vi "pueba.vi"(0 "Ruta":path, 3 "Método":enum16{"G", "Gx", "Gy"}(ring)) -> ()   [LabVIEW 2020]
doc: "Ceballos Conde Emanuel 4MV6 Sistemas de visión artificial 2022/1\nEste vi permite obtener el gradiente en x , gradiente en Y o gradiente general en susecion de una serie de imagenes ubicadas en una carpeta , si se utiliza como subvi la salida obtenida sera el gradiente da la ultima imagen de la carpeta."
panel:
  out "Bcx":u32
  out "Bcy":u32
  out "Gcx":u32
  out "Gcy":u32
  out "Rcy":u32
  out "Rcx":u32
  out "Image":T1(plugin-control)
  # "Ceballos Conde Emanuel\n4MV6\nSistemas de visión artificial\n2022/1"
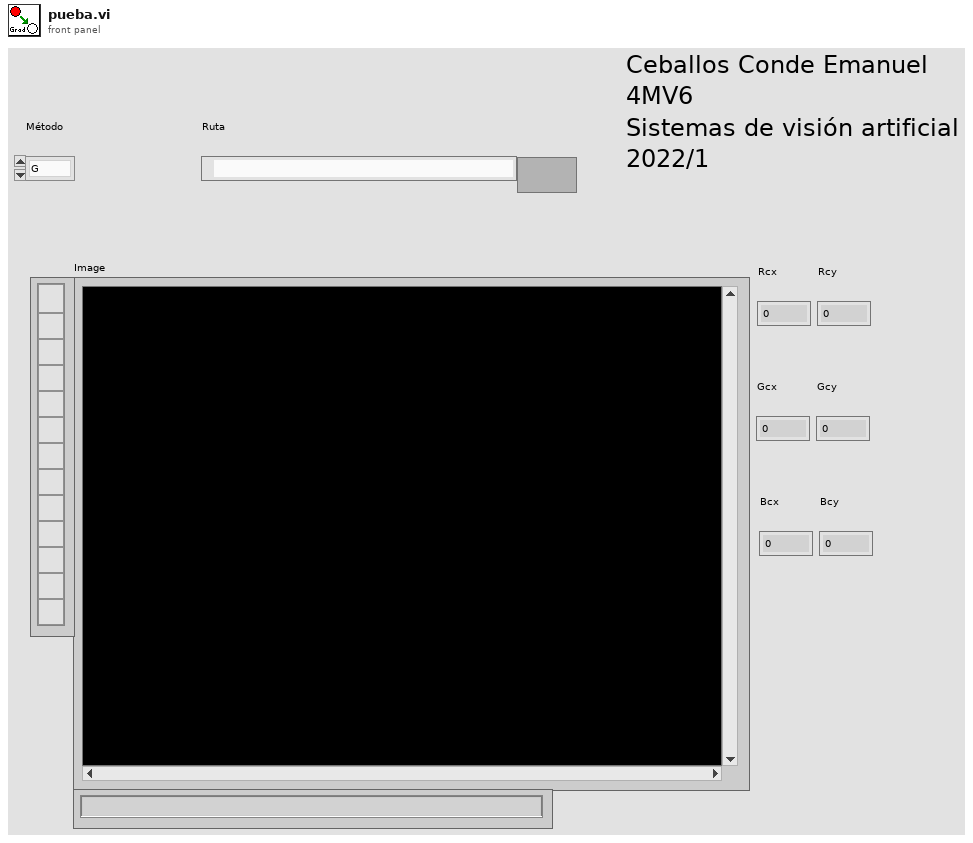
[diagram p1: front panel]
types:
  T1 = typedef "IMAQ Image.ctl" = refnum<image>
  T2 = typedef "Image Type" = u32
  T3 = typedef "imagedata.ctl" = cluster{"image type":i32, "image depth":i32, "image":u8[], "mask":u8[], "colors":u32[], "Rectangle":cluster{"left":i16, "top":i16, "right":i16, "bottom":i16}}
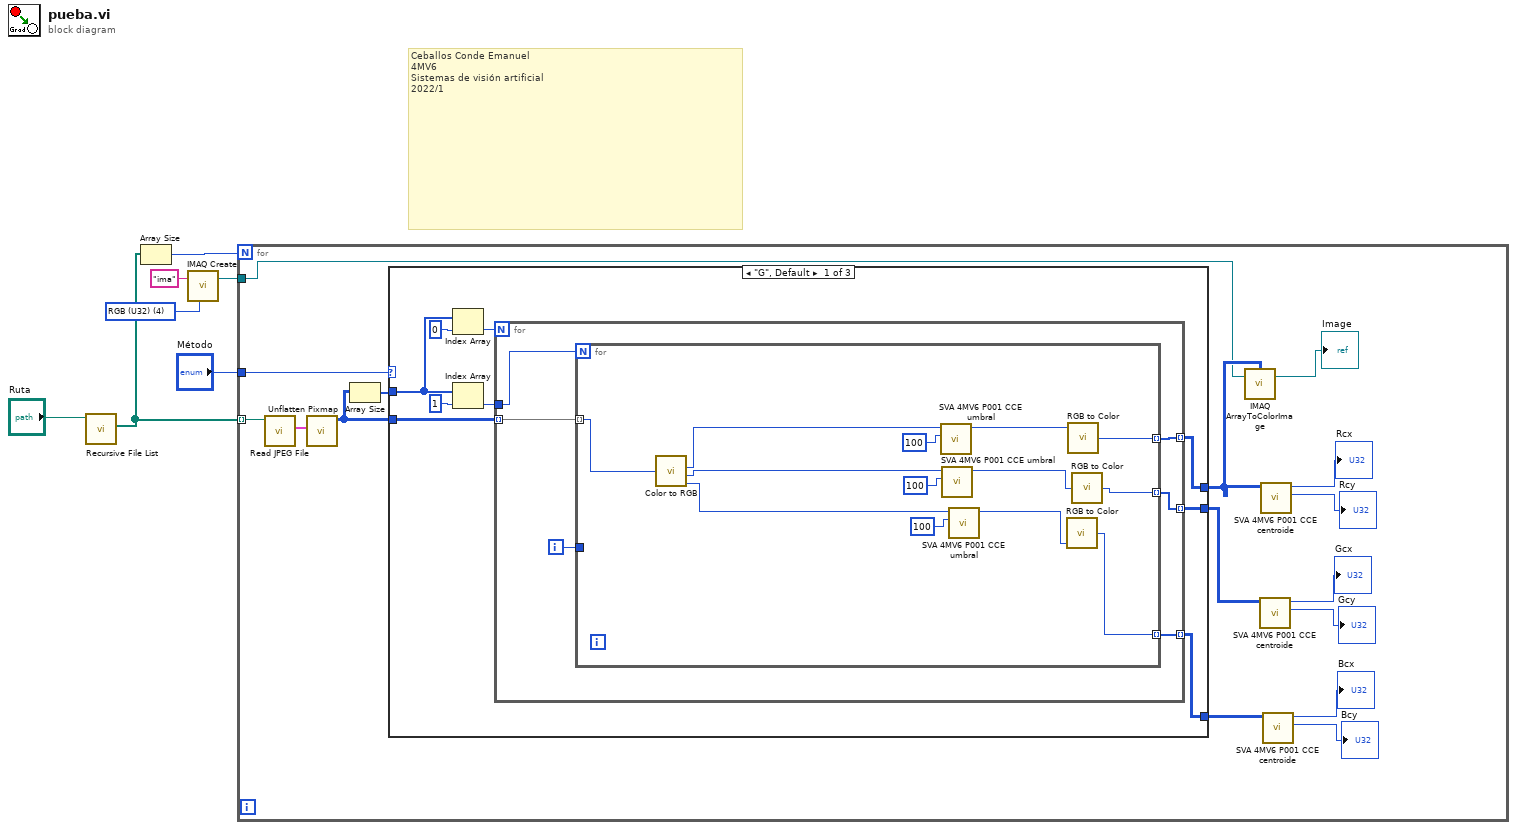
[diagram p0: block diagram]
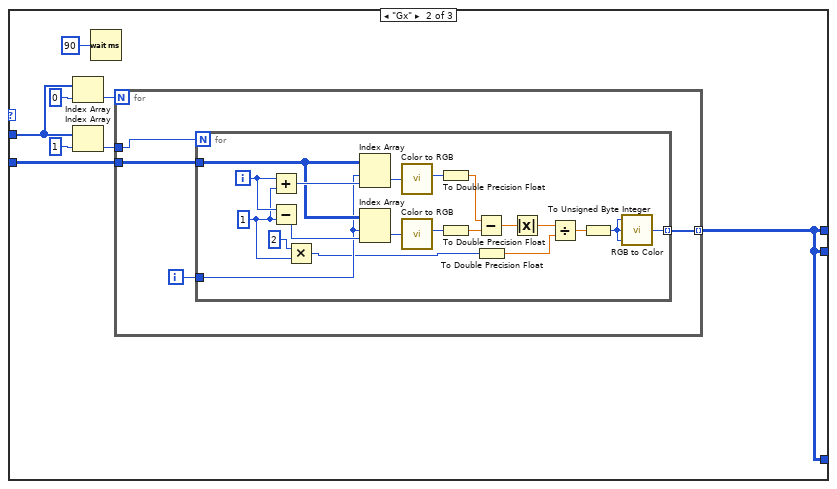
[diagram p2: hidden frame]
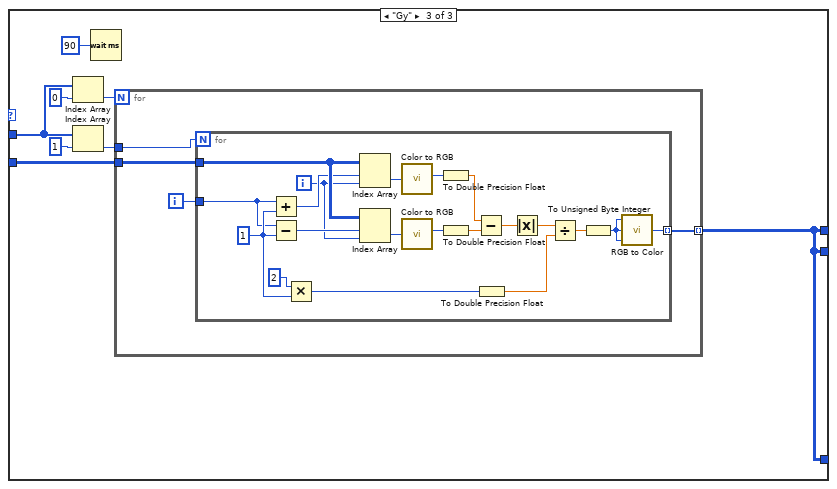
[diagram p3: hidden frame]
diagram:
  w1 = T2 4 items=["Grayscale (U8)", "Grayscale (I16)", "Grayscale (SGL)", "Complex (CSG)", "RGB (U32)", "HSL (U32)", "RGB (U64)", "Grayscale (U16)"] ("Image Type")
  # "Ceballos Conde Emanuel\n4MV6\nSistemas de visión artificial\n2022/1"
  n1 = call <vilib>:"Recursive File List.vi"("Folder Path"="Ruta") -> ("All Files in Dir"=w7:path[])  [unwired: 6 in, 4 out]
  n2 = Array Size(array=w7) -> (size(s)=w6:i32)
  n3 = call "IMAQ Create"("Image Name"="ima", "Image Type"=w1) -> ("New Image"=w3:T1)  [unwired: 3 in, 1 out]
  n4 = for {
    N: w6 -> [_]
    tunnel: w7 -> [w20] mode=indexing
    tunnel: "Método" -> [w19]
    tunnel: w3 -> [w14]
    n5 = call <vilib>:"Read JPEG File.vi"("path to JPEG file"=w20) -> ("image data"=w23:T3)  [unwired: 8 in, 2 out]
    n6 = call <vilib>:"Unflatten Pixmap.vi"("image data"=w23) -> ("24-bit pixmap"=w22:u32[][])  [unwired: 4 in, 6 out]
    n7 = Array Size(array=w22) -> (size(s)=w21:i32[])
    n8 = case shown="\"G\", Default" w19 {
      tunnel: w22 -> [w27 w59 w87]
      tunnel: [w28 w52 w84] -> w17
      tunnel: w21 -> [w26 w55 w86]
      tunnel: [w25 w52 w84] -> w9
      tunnel: [w24 w52 w84] -> w8
      frame "G", Default {
        n9 = Index Array(array=w26, index=0) -> (element=w32:i32)
        n10 = Index Array(array=w26, index=1) -> (element=w30:i32)
        n11 = for {
          N: w32 -> [_]
          tunnel: w27 -> [w38] mode=indexing
          tunnel: [w36] -> w28 mode=indexing
          tunnel: w30 -> [w35]
          tunnel: [w34] -> w25 mode=indexing
          tunnel: [w33] -> w24 mode=indexing
          i -> [w37]
          n12 = for {
            N: w35 -> [_]
            tunnel: w38 -> [w51] mode=indexing
            tunnel: w37 -> [_]
            tunnel: [w43] -> w36 mode=indexing
            tunnel: [w40] -> w34 mode=indexing
            tunnel: [w39] -> w33 mode=indexing
            n13 = call <vilib>:"Color to RGB.vi"("Color"=w51) -> ("R"=w45:u8, "G"=w46:u8, "B"=w49:u8)  [unwired: 1 out]
            n14 = call "SVA 4MV6 P001 CCE umbral.vi"("gris"=w45, "umbral"=u8 100) -> ("umbralizado"=w44:u8)  [unwired: 8 in]
            n15 = call "SVA 4MV6 P001 CCE umbral.vi"("gris"=w46, "umbral"=u8 100) -> ("umbralizado"=w42:u8)  [unwired: 8 in]
            n16 = call "SVA 4MV6 P001 CCE umbral.vi"("gris"=w49, "umbral"=u8 100) -> ("umbralizado"=w41:u8)  [unwired: 8 in]
            n17 = call <vilib>:"RGB to Color.vi"("B"=w41) -> ("Color"=w39:u32)  [unwired: 2 in]
            n18 = call <vilib>:"RGB to Color.vi"("R"=w44) -> ("Color"=w43:u32)  [unwired: 2 in]
            n19 = call <vilib>:"RGB to Color.vi"("G"=w42) -> ("Color"=w40:u32)  [unwired: 2 in]
          }
        }
      }
      frame "Gx" {
        n20 = Index Array(array=w55, index=0) -> (element=w58:i32)
        n21 = Index Array(array=w55, index=1) -> (element=w56:i32)
        n22 = Wait (ms)(milliseconds to wait=u32 90) -> ()  [unwired: 1 out]
        n23 = for {
          N: w58 -> [_]
          tunnel: w59 -> [w63]
          tunnel: [w61] -> w52 mode=indexing
          tunnel: w56 -> [w60]
          i -> [w62]
          n24 = for {
            N: w60 -> [_]
            tunnel: w63 -> [w78]
            tunnel: w62 -> [w77]
            tunnel: [w79] -> w61 mode=indexing
            i -> [w76]
            w71 = 1
            n25 = Add(x=w76, y=w71) -> (x+y=w81:i32)
            n26 = Subtract(x=w76, y=w71) -> (x-y=w80:i32)
            n27 = Multiply(x=2, y=w71) -> (x*y=w72:i32)
            n28 = Index Array(array=w78, index (row)=w77, index (col)=w81) -> (element=w83:u32)
            n29 = Index Array(array=w78, index (row)=w77, index (col)=w80) -> (element=w82:u32)
            n30 = call <vilib>:"Color to RGB.vi"("Color"=w83) -> ("R"=w75:u8)  [unwired: 3 out]
            n31 = call <vilib>:"Color to RGB.vi"("Color"=w82) -> ("R"=w74:u8)  [unwired: 3 out]
            n32 = To Double Precision Float(number=w75) -> (double precision float=w67:dbl)
            n33 = To Double Precision Float(number=w74) -> (double precision float=w66:dbl)
            n34 = Subtract(x=w67, y=w66) -> (x-y=w73:dbl)
            n35 = To Double Precision Float(number=w72) -> (double precision float=w65:dbl)
            n36 = Absolute Value(x=w73) -> (abs(x)=w68:dbl)
            n37 = Divide(x=w68, y=w65) -> (x/y=w69:dbl)
            n38 = To Unsigned Byte Integer(number=w69) -> (unsigned 8bit integer=w64:u8)
            n39 = call <vilib>:"RGB to Color.vi"("B"=w64, "G"=w64, "R"=w64) -> ("Color"=w79:u32)
          }
        }
      }
      frame "Gy" {
        n40 = Index Array(array=w86, index=0) -> (element=w90:i32)
        n41 = Index Array(array=w86, index=1) -> (element=w91:i32)
        n42 = Wait (ms)(milliseconds to wait=u32 90) -> ()  [unwired: 1 out]
        n43 = for {
          N: w90 -> [_]
          tunnel: w87 -> [w95]
          tunnel: [w93] -> w84 mode=indexing
          tunnel: w91 -> [w92]
          i -> [w94]
          n44 = for {
            N: w92 -> [_]
            tunnel: w95 -> [w112]
            tunnel: w94 -> [w97]
            tunnel: [w113] -> w93 mode=indexing
            i -> [w96]
            w107 = 1
            n45 = Add(x=w97, y=w107) -> (x+y=w99:i32)
            n46 = Subtract(x=w97, y=w107) -> (x-y=w98:i32)
            n47 = Multiply(x=2, y=w107) -> (x*y=w108:i32)
            n48 = Index Array(array=w112, index (row)=w99, index (col)=w96) -> (element=w115:u32)
            n49 = Index Array(array=w112, index (row)=w98, index (col)=w96) -> (element=w114:u32)
            n50 = call <vilib>:"Color to RGB.vi"("Color"=w115) -> ("R"=w111:u8)  [unwired: 3 out]
            n51 = call <vilib>:"Color to RGB.vi"("Color"=w114) -> ("R"=w110:u8)  [unwired: 3 out]
            n52 = To Double Precision Float(number=w111) -> (double precision float=w103:dbl)
            n53 = To Double Precision Float(number=w110) -> (double precision float=w102:dbl)
            n54 = Subtract(x=w103, y=w102) -> (x-y=w109:dbl)
            n55 = To Double Precision Float(number=w108) -> (double precision float=w101:dbl)
            n56 = Absolute Value(x=w109) -> (abs(x)=w104:dbl)
            n57 = Divide(x=w104, y=w101) -> (x/y=w105:dbl)
            n58 = To Unsigned Byte Integer(number=w105) -> (unsigned 8bit integer=w100:u8)
            n59 = call <vilib>:"RGB to Color.vi"("B"=w100, "G"=w100, "R"=w100) -> ("Color"=w113:u32)
          }
        }
      }
    }
    n60 = call "IMAQ ArrayToColorImage"("Image Pixels (U32)"=w17, "Image"=w14) -> ("Image Out"=→"Image":T1)  [unwired: 3 in, 1 out]
    n61 = call "SVA 4MV6 P001 CCE centroide .vi"("Array"=w9) -> ("cy"=→"Gcy":u32, "cx"=→"Gcx":u32)  [unwired: 9 in]
    n62 = call "SVA 4MV6 P001 CCE centroide .vi"("Array"=w17) -> ("cy"=→"Rcy":u32, "cx"=→"Rcx":u32)  [unwired: 9 in]
    n63 = call "SVA 4MV6 P001 CCE centroide .vi"("Array"=w8) -> ("cy"=→"Bcy":u32, "cx"=→"Bcx":u32)  [unwired: 9 in]
  }
